vi "Get Sessions Info Impl.vi"(8 "error in":errorcluster, 11 "session reservation in":refnum<class "Session Reservation.lvclass">) -> (0 "error out":errorcluster, 2 "sessions info":T1[](array[typedef]), 3 "session reservation out":refnum<class "Session Reservation.lvclass">)   [LabVIEW 2020, in "MeasurementLink Session Management.lvlib" / "Session Reservation.lvclass"]
doc: "Gets the connection information for the given <b>pin type</b>, <b>pin or relay name</b>, <b>instrument</b>, and <b>site</b>.The <b>instrument</b> input must return a valid instrument_type_id from the <b>Get Instrument Type ID.vi</b> override. The <b>connection type</b> input should be a cluster with two elements. The first element is a <b>Connection.ctl</b> cluster. The second element is the type of the session."
uses:
  Session Reservation.lvclass
  MeasurementLink Session Management Client/RPC Messages/ni_measurementlink_sessionmanagement_v1_SessionInformation.ctl
  MeasurementLink Session Management Client/RPC Messages/nidevice_grpc_Session.ctl
  MeasurementLink Session Management Client/RPC Messages/ni_measurementlink_sessionmanagement_v1_ChannelMapping.ctl
  Session Reservation.lvclass/Session Reservation.ctl
  MeasurementLink Measurement Server/Helpers/Error Strings Global Internal.vi
  MeasurementLink Session Management Client/MeasurementLink Session Management Client.lvlib
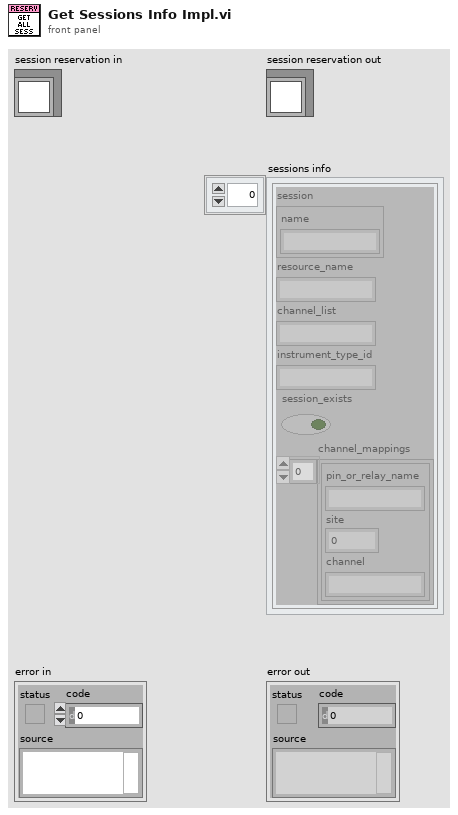
[diagram p1: front panel]
types:
  T1 = typedef "MeasurementLink Session Management Client.lvlib/ni_measurementlink_sessionmanagement_v1_SessionInformation.ctl" = cluster{"session":T2, "resource_name":string, "channel_list":string, "instrument_type_id":string, "session_exists":bool, "channel_mappings":T3[]}
  T2 = typedef "MeasurementLink Session Management Client.lvlib/nidevice_grpc_Session.ctl" = cluster{"name":string}
  T3 = typedef "MeasurementLink Session Management Client.lvlib/ni_measurementlink_sessionmanagement_v1_ChannelMapping.ctl" = cluster{"pin_or_relay_name":string, "site":i32, "channel":string}
  T4 = typedef "MeasurementLink Session Management.lvlib/Session Reservation.lvclass/Data.ctl" = cluster{"session and driver infos":T5[], "pin or relay names":string[], "connection map":refnum<class "Connection Map.lvclass">, "pin map context":T6, "reservation observer":refnum<class "IReservationObserver.lvclass">, "dvr valid":bool}
  T5 = typedef "MeasurementLink Session Management.lvlib/Session Reservation.lvclass/Session and Driver Info.ctl" = cluster{"session info":T1, "session":variant, "instrument":refnum<class "IInstrument.lvclass">}
  T6 = typedef "MeasurementLink Session Management Client.lvlib/ni_measurementlink_PinMapContext.ctl" = cluster{"pin_map_id":string, "sites":i32[]}
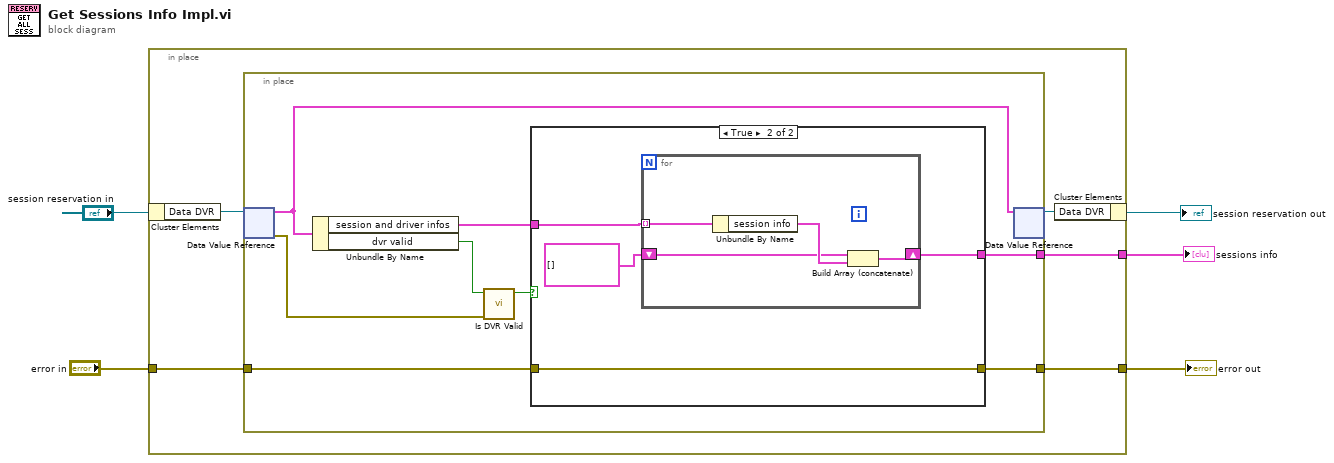
[diagram p0: block diagram]
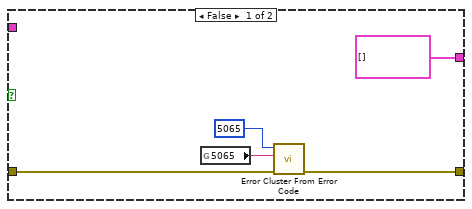
[diagram p2: hidden frame]
diagram:
  n1 = in-place {
    in-place-border: "error in" -> [w10]
    in-place-border: [w9] -> w1
    in-place-border: [w6] -> w5
    n2 = in-place-cluster #1("session reservation in") -> ("Data DVR"=w8:refnum<data-value>)
    n3 = in-place {
      in-place-border: w10 -> [w18]
      in-place-border: [w17] -> w9
      in-place-border: [w14] -> w6
      n4 = in-place-dvr #2(w8) -> (w15:T4, w11:errorcluster)
      n5 = Unbundle By Name(w15) -> ("session and driver infos"=w16:T5[], "dvr valid"=w13:bool)
      n6 = call "Is DVR Valid.vi"("dvr error in"=w11, "dvr valid"=w13) -> ("dvr valid"=w12:bool)  [unwired: 9 in]
      n7 = case shown="True" w12 {
        tunnel: w18 -> [w21 w27]
        tunnel: [w20 w27] -> w17
        tunnel: w16 -> [_ w26]
        tunnel: [T1[] [] w24] -> w14
        frame False {
          n8 = global read "Error Strings Global Internal.vi" "5065"() -> (w23:string)
          n9 = call <vilib>:"Error Cluster From Error Code.vi"("error in (no error)"=w21, "error message (\"\")"=w23, "error code (0)"=5065) -> ("error out"=w20:errorcluster)  [unwired: 6 in]
        }
        frame True {
          n10 = for {
            tunnel: w26 -> [w31] mode=indexing
            shift-right: [w28] -> w24
            shift-left: T1[] [] -> [w29]
            n11 = Unbundle By Name(w31) -> ("session info"=w30:T1)
            n12 = Build Array (concatenate)(w29, w30) -> (w28:T1[])
          }
        }
      }
      n13 = in-place-dvr #2(w15) -> (w7:refnum<data-value>)  [unwired: 1 out]
    }
    n14 = in-place-cluster #1("Data DVR"=w7) -> (→"session reservation out":refnum<class "Session Reservation.lvclass">)
  }
  "error out" <- w1
  "sessions info" <- w5
